vi "Y1AndY2.vi"(0 "Cam 0":T2={"position"=0.0, "pixelsize"=0.0, "start"=0.0, "end"=0.0, "center"=0.0, "Lens"=enum."FL1-f8x08", "Forward"=enum."off", "Spec_Calib_file 2"=path "Y:/100TWdata/ESMCalib/datFwd.txt", "map"=path "Y:/100TWdata/ESMCalib/mapFwd.txt", "y size"=0, "UserROI"={"Width"={"Value"=0.0, "Min"=0.0, "Max"=0.0, "StepSize"=0.0, "Tolerance"=0.0, "ValueActual"=0.0}, "Hight"={"Value"=0.0, "Min"=0.0, "Max"=0.0, "StepSize"=0.0, "Tolerance"=0.0, "ValueActual"=0.0}, "OffsetX"={"Value"=0.0, "Min"=0.0, "Max"=0.0, "StepSize"=0.0, "Tolerance"=0.0, "ValueActual"=0.0}, "OffsetY"={"Value"=0.0, "Min"=0.0, "Max"=0.0, "StepSize"=0.0, "Tolerance"=0.0, "ValueActual"=0.0}}, "CamMaxPixel"={"X"=0, "Y"=0}, "CamROI"={"Width"=0.0, "Hight"=0.0, "OffsetX"=0.0, "OffsetY"=0.0}}, 5 "Cluster":T8, 9 "position":dbl) -> (4 "Cam 1":T2={"position"=0.0, "pixelsize"=0.0, "start"=0.0, "end"=0.0, "center"=0.0, "Lens"=enum."FL1-f8x08", "Forward"=enum."off", "Spec_Calib_file 2"=path "Y:/100TWdata/ESMCalib/datFwd.txt", "map"=path "Y:/100TWdata/ESMCalib/mapFwd.txt", "y size"=0, "UserROI"={"Width"={"Value"=0.0, "Min"=0.0, "Max"=0.0, "StepSize"=0.0, "Tolerance"=0.0, "ValueActual"=0.0}, "Hight"={"Value"=0.0, "Min"=0.0, "Max"=0.0, "StepSize"=0.0, "Tolerance"=0.0, "ValueActual"=0.0}, "OffsetX"={"Value"=0.0, "Min"=0.0, "Max"=0.0, "StepSize"=0.0, "Tolerance"=0.0, "ValueActual"=0.0}, "OffsetY"={"Value"=0.0, "Min"=0.0, "Max"=0.0, "StepSize"=0.0, "Tolerance"=0.0, "ValueActual"=0.0}}, "CamMaxPixel"={"X"=0, "Y"=0}, "CamROI"={"Width"=0.0, "Hight"=0.0, "OffsetX"=0.0, "OffsetY"=0.0}}, 6 "Clustero ut":T8, 8 "calib(pixel)":T1, 10 "position 2":dbl)   [LabVIEW 2013]
uses:
  configTypDEf.ctl
  CamSettingSUB_TypDEf.ctl
  MagAnalysis_Online_Bella/SubVis/CamAndObj_TypDEf.ctl
  shared/OnOffTypeDef.ctl
  userROI.ctl
  shared/numericVariable_TypeDef.ctl
  CamRoiTypDef.ctl
  calibPixel.ctl
  BaseDriver/BaseDriver.lvclass
panel:
  out "y1":dbl[](array[numeric])
  out "y2":dbl[](array[numeric])
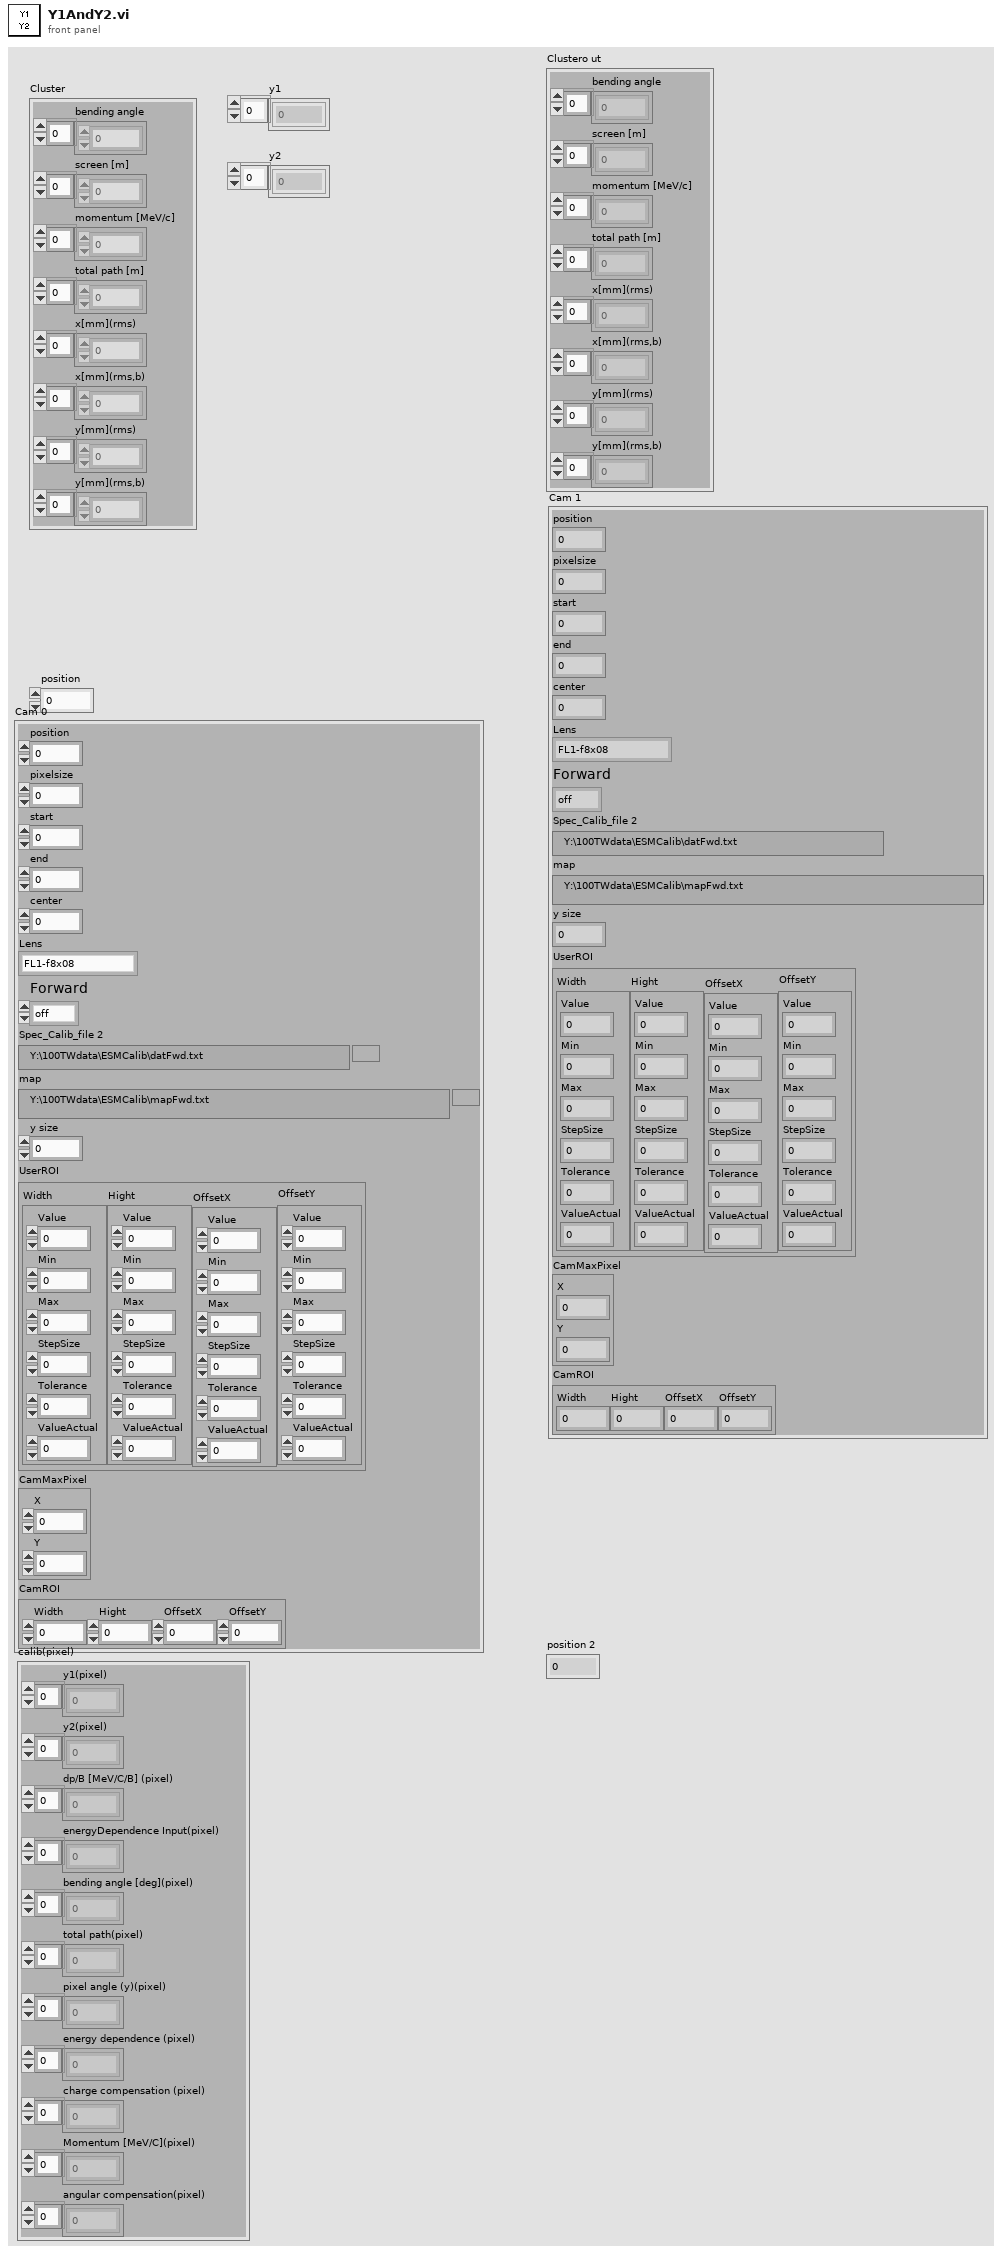
[diagram p1: front panel]
types:
  T1 = typedef "calibPixel.ctl" = cluster{"y1(pixel)":dbl[], "y2(pixel)":dbl[], "dp/B [MeV/C/B] (pixel)":dbl[], "energyDependence Input(pixel)":dbl[], "bending angle [deg](pixel)":dbl[], "total path(pixel)":dbl[], "pixel angle (y)(pixel)":dbl[], "energy dependence (pixel)":dbl[], "charge compensation (pixel)":dbl[], "Momentum [MeV/C](pixel)":dbl[], "angular compensation(pixel)":dbl[]}
  T2 = typedef "CamSettingSUB_TypDEf.ctl" = cluster{"position":dbl, "pixelsize":dbl, "start":dbl, "end":dbl, "center":dbl, "Lens":T3, "Forward":T4, "Spec_Calib_file 2":path, "map":path, "y size":i32, "UserROI":T5, "CamMaxPixel":cluster{"X":i32, "Y":i32}, "CamROI":T7}
  T3 = typedef "CamAndObj_TypDEf.ctl" = enum16{"FL1-f8x08", "FL1-f8x06", "FL1-f8", "ch300-f50", "FL2G-f8", "FL3M14-f8", "FL3M14-f8x08", "FL3M14-f8x08(2x2)"}
  T4 = typedef "OnOffTypeDef.ctl" = enum16{"off", "on"}
  T5 = typedef "userROI.ctl" = cluster{"Width":T6, "Hight":T6, "OffsetX":T6, "OffsetY":T6}
  T6 = typedef "BaseDriver.lvclass/numericVariable_TypeDef.ctl" = cluster{"Value":dbl, "Min":dbl, "Max":dbl, "StepSize":dbl, "Tolerance":dbl, "ValueActual":dbl}
  T7 = typedef "CamRoiTypDef.ctl" = cluster{"Width":dbl, "Hight":dbl, "OffsetX":dbl, "OffsetY":dbl}
  T8 = typedef "configTypDEf.ctl" = cluster{"bending angle":dbl[], "screen [m]":dbl[], "momentum [MeV/c]":dbl[], "total path [m]":dbl[], "x[mm](rms)":dbl[], "x[mm](rms,b)":dbl[], "y[mm](rms)":dbl[], "y[mm](rms,b)":dbl[]}
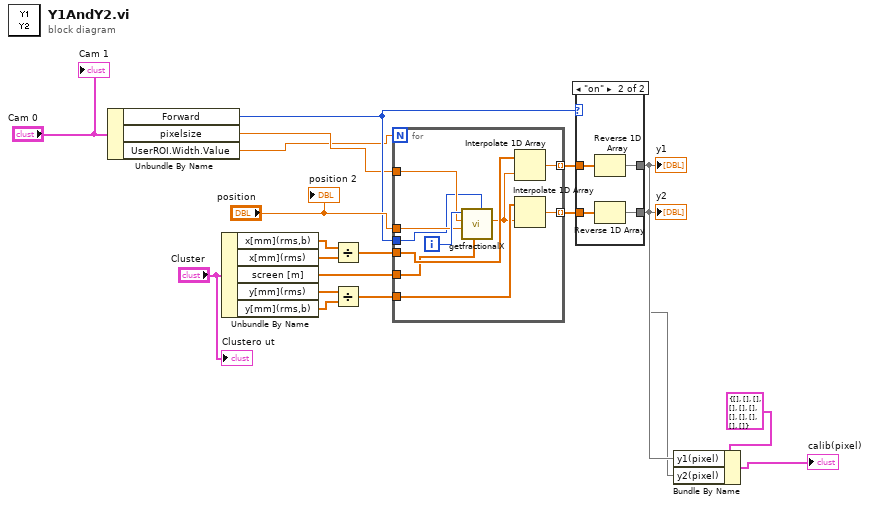
[diagram p0: block diagram]
diagram:
  n1 = Unbundle By Name("Cam 0") -> ("Forward"=w7:T4, "pixelsize"=w6:dbl, "UserROI.Width.Value"=w5:dbl)
  n2 = Unbundle By Name("Cluster") -> ("x[mm](rms,b)"=w15:dbl[], "x[mm](rms)"=w16:dbl[], "screen [m]"=w10:dbl[], "y[mm](rms)"=w12:dbl[], "y[mm](rms,b)"=w13:dbl[])
  n3 = Divide(x=w15, y=w16) -> (x/y=w17:dbl[])
  n4 = Divide(x=w12, y=w13) -> (x/y=w14:dbl[])
  n5 = for {
    N: w5 -> [_]
    tunnel: w10 -> [w22]
    tunnel: w6 -> [w24]
    tunnel: "position" -> [w23]
    tunnel: w17 -> [w29]
    tunnel: w14 -> [w28]
    tunnel: [w27] -> w18 mode=indexing
    tunnel: [w26] -> w19 mode=indexing
    tunnel: w7 -> [w20]
    i -> [w25]
    n6 = call "getfractionalX.vi"("forward"=w20, "screen [m]"=w22, "position"=w23, "pixelsize"=w24, "Numeric in"=w25) -> ("index"=w21:dbl)  [unwired: 5 in, 1 out]
    n7 = Interpolate 1D Array(1:w21, 2:w29) -> (0:w27:dbl)
    n8 = Interpolate 1D Array(1:w21, 2:w28) -> (0:w26:dbl)
  }
  n9 = case shown="\"on\"" w7 {
    tunnel: [w30 w35] -> w3
    tunnel: w18 -> [w30 w34]
    tunnel: [w31 w33] -> w2
    tunnel: w19 -> [w31 w32]
    frame "off", Default {
    }
    frame "on" {
      n10 = Reverse 1D Array(array=w34) -> (reversed array=w35:dbl[])
      n11 = Reverse 1D Array(array=w32) -> (reversed array=w33:dbl[])
    }
  }
  "y2" <- w2
  "y1" <- w3
  n12 = Bundle By Name(cluster=T1 {"y1(pixel)"=[], "y2(pixel)"=[], "dp/B [MeV/C/B] (pixel)"=[], "energyDependence Input(pixel)"=[], "bending angle [deg](pixel)"=[], "total path(pixel)"=[], "pixel angle (y)(pixel)"=[], "energy dependence (pixel)"=[], "charge compensation (pixel)"=[], "Momentum [MeV/C](pixel)"=[], "angular compensation(pixel)"=[]}, "y1(pixel)"=w3, "y2(pixel)"=w2) -> (→"calib(pixel)":T1)
  "Clustero ut" <- "Cluster"
  "Cam 1" <- "Cam 0"
  "position 2" <- "position"
